vi "参数配置表.vi"() -> ()   [LabVIEW 2016, in "数据传输系统.lvlib"]
uses:
  <vilib>/Utility/miscctls.llb/LVPointTypeDef.ctl
  <vilib>/ptbypt/NI_PtbyPt.lvlib
panel:
  in  "协议标准":T1(ring)
  in  "加密传输":bool
  in  "数据库类型":enum16{"Access", "SQLite"}(ring)
  in  "应用环境":T2
  in  "屏蔽维护数据":bool
  in  "数据发送延时时间/s":i32
  in  "判断数据反馈":enum16{"非严格判断", "严格判断", "不判断"}(ring)
  in  "仪器参数发送":bool
  in  "地表水/污染源":bool
  in  "间隔时间/分钟":i32
  in  "数据发送通道":enum16{"TCP", "VISA"}(ring)
  in  "数据发送协议":enum16{"2005-212协议", "2017-212协议"}(ring)=enum."2017-212协议"
  in  "数据触发上传方式":enum16{"出数即刻发送", "间隔时间发送", "整点发送"}(ring)
  in  "数据组合发送":bool
  in  "日志、参数发送":bool
  in  "2011发送":bool
  in  "返回":bool
  out "配置表格":string[][](table)
  in  "参数数值":T3={"CODMn"=TRUE, "CODCr"=TRUE, "DO"=TRUE, "铜"=TRUE, "PH"=TRUE, "氨氮"=TRUE, "比电导率"=TRUE, "水温"=TRUE, "COD"=TRUE, "浊度"=TRUE, "总氮"=TRUE, "总磷"=TRUE, "叶绿素a"=TRUE, "藻密度"=TRUE, "水位"=TRUE, "流速"=TRUE, "瞬时流量"=TRUE, "累积流量"=TRUE, "亚硝氮"=TRUE, "硫化物"=TRUE, "ORP"=TRUE, "铅"=TRUE, "镉"=TRUE, "锌"=TRUE, "镍"=TRUE, "锰"=TRUE, "汞"=TRUE, "气温"=TRUE, "气压"=TRUE, "风速"=TRUE, "风向"=TRUE, "盐度"=TRUE, "磷酸盐"=TRUE, "硝氮"=TRUE, "氟化物"=TRUE, "挥发酚"=TRUE, "氯化物"=TRUE, "蓝绿藻"=TRUE}
  # "因子编码，单位配置，上传功能码，小时、质控数据上传触发方式"
  # "参数配置"
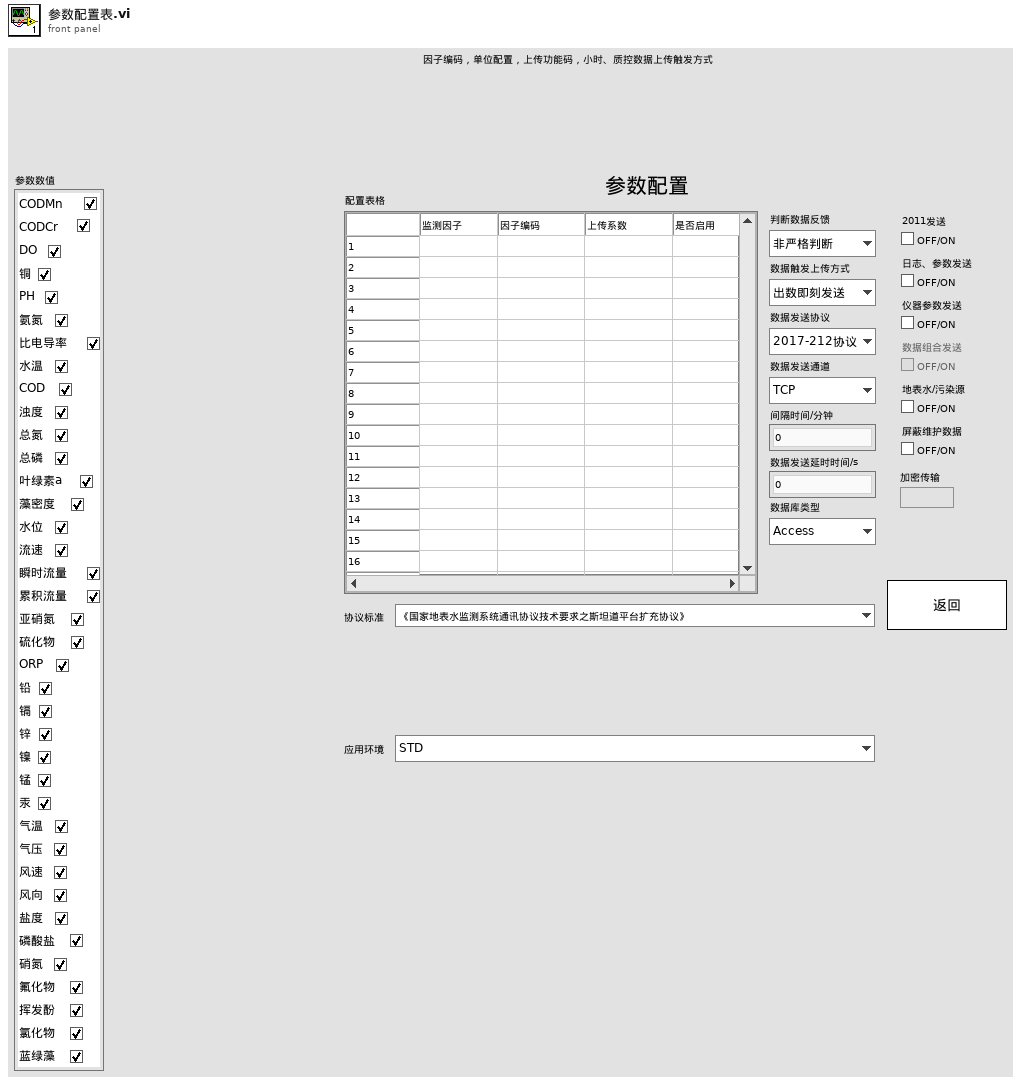
[diagram p1: front panel]
types:
  T1 = enum16{"《国家地表水监测系统通讯协议技术要求之斯坦道平台扩充协议》", "《国家地表水监测系统通讯协议技术要求》", "《国家地表水监测系统通讯协议技术要求之安徽皖仪省级平台扩充协议》"}
  T2 = typedef "数据传输系统.lvlib/应用环境.ctl" = enum16{"STD", "GB212", "婉仪平台"}
  T3 = cluster{"CODMn":bool, "CODCr":bool, "DO":bool, "铜":bool, "PH":bool, "氨氮":bool, "比电导率":bool, "水温":bool, "COD":bool, "浊度":bool, "总氮":bool, "总磷":bool, "叶绿素a":bool, "藻密度":bool, "水位":bool, "流速":bool, "瞬时流量":bool, "累积流量":bool, "亚硝氮":bool, "硫化物":bool, "ORP":bool, "铅":bool, "镉":bool, "锌":bool, "镍":bool, "锰":bool, "汞":bool, "气温":bool, "气压":bool, "风速":bool, "风向":bool, "盐度":bool, "磷酸盐":bool, "硝氮":bool, "氟化物":bool, "挥发酚":bool, "氯化物":bool, "蓝绿藻":bool}
  T4 = typedef "LVPointTypeDef.ctl" = cluster{"Horizontal":i16, "Vertical":i16}
  T5 = cluster{"[0]":string, "[1]":string, "[2]":string, "[3]":string, "[4]":string, "[5]":string, "[6]":string, "[7]":string, "[8]":string, "[9]":string, "[10]":string, "[11]":string, "[12]":string, "[13]":string, "[14]":string, "[15]":string, "[16]":string, "[17]":string, "[18]":string, "[19]":string, "[20]":string, "[21]":string, "[22]":string, "[23]":string, "[24]":string, "[25]":string, "[26]":string, "[27]":string, "[28]":string, "[29]":string, "[30]":string, "[31]":string, "[32]":string, "[33]":string, "[34]":string, "[35]":string, "[36]":string, "[37]":string}
  T6 = enum8{"Enabled", "Disabled", "Disabled and Grayed Out"}
  T7 = typedef "LVRowAndColumnTypeDef.ctl" = cluster{"Row":i32, "Column":i32}
  T8 = cluster{"[0]":string, "[1]":string, "[2]":string, "[3]":string, "[4]":string, "[5]":string, "[6]":string, "[7]":string}
  T9 = cluster{"[0]":string, "[1]":string, "[2]":string, "[3]":string, "[4]":string, "[5]":string, "[6]":string, "[7]":string, "[8]":string, "[9]":string, "[10]":string, "[11]":string, "[12]":string, "[13]":string}
  T10 = cluster{"[0]":string, "[1]":string, "[2]":string, "[3]":string, "[4]":string, "[5]":string, "[6]":string, "[7]":string, "[8]":string, "[9]":string, "[10]":string, "[11]":string, "[12]":string, "[13]":string, "[14]":string}
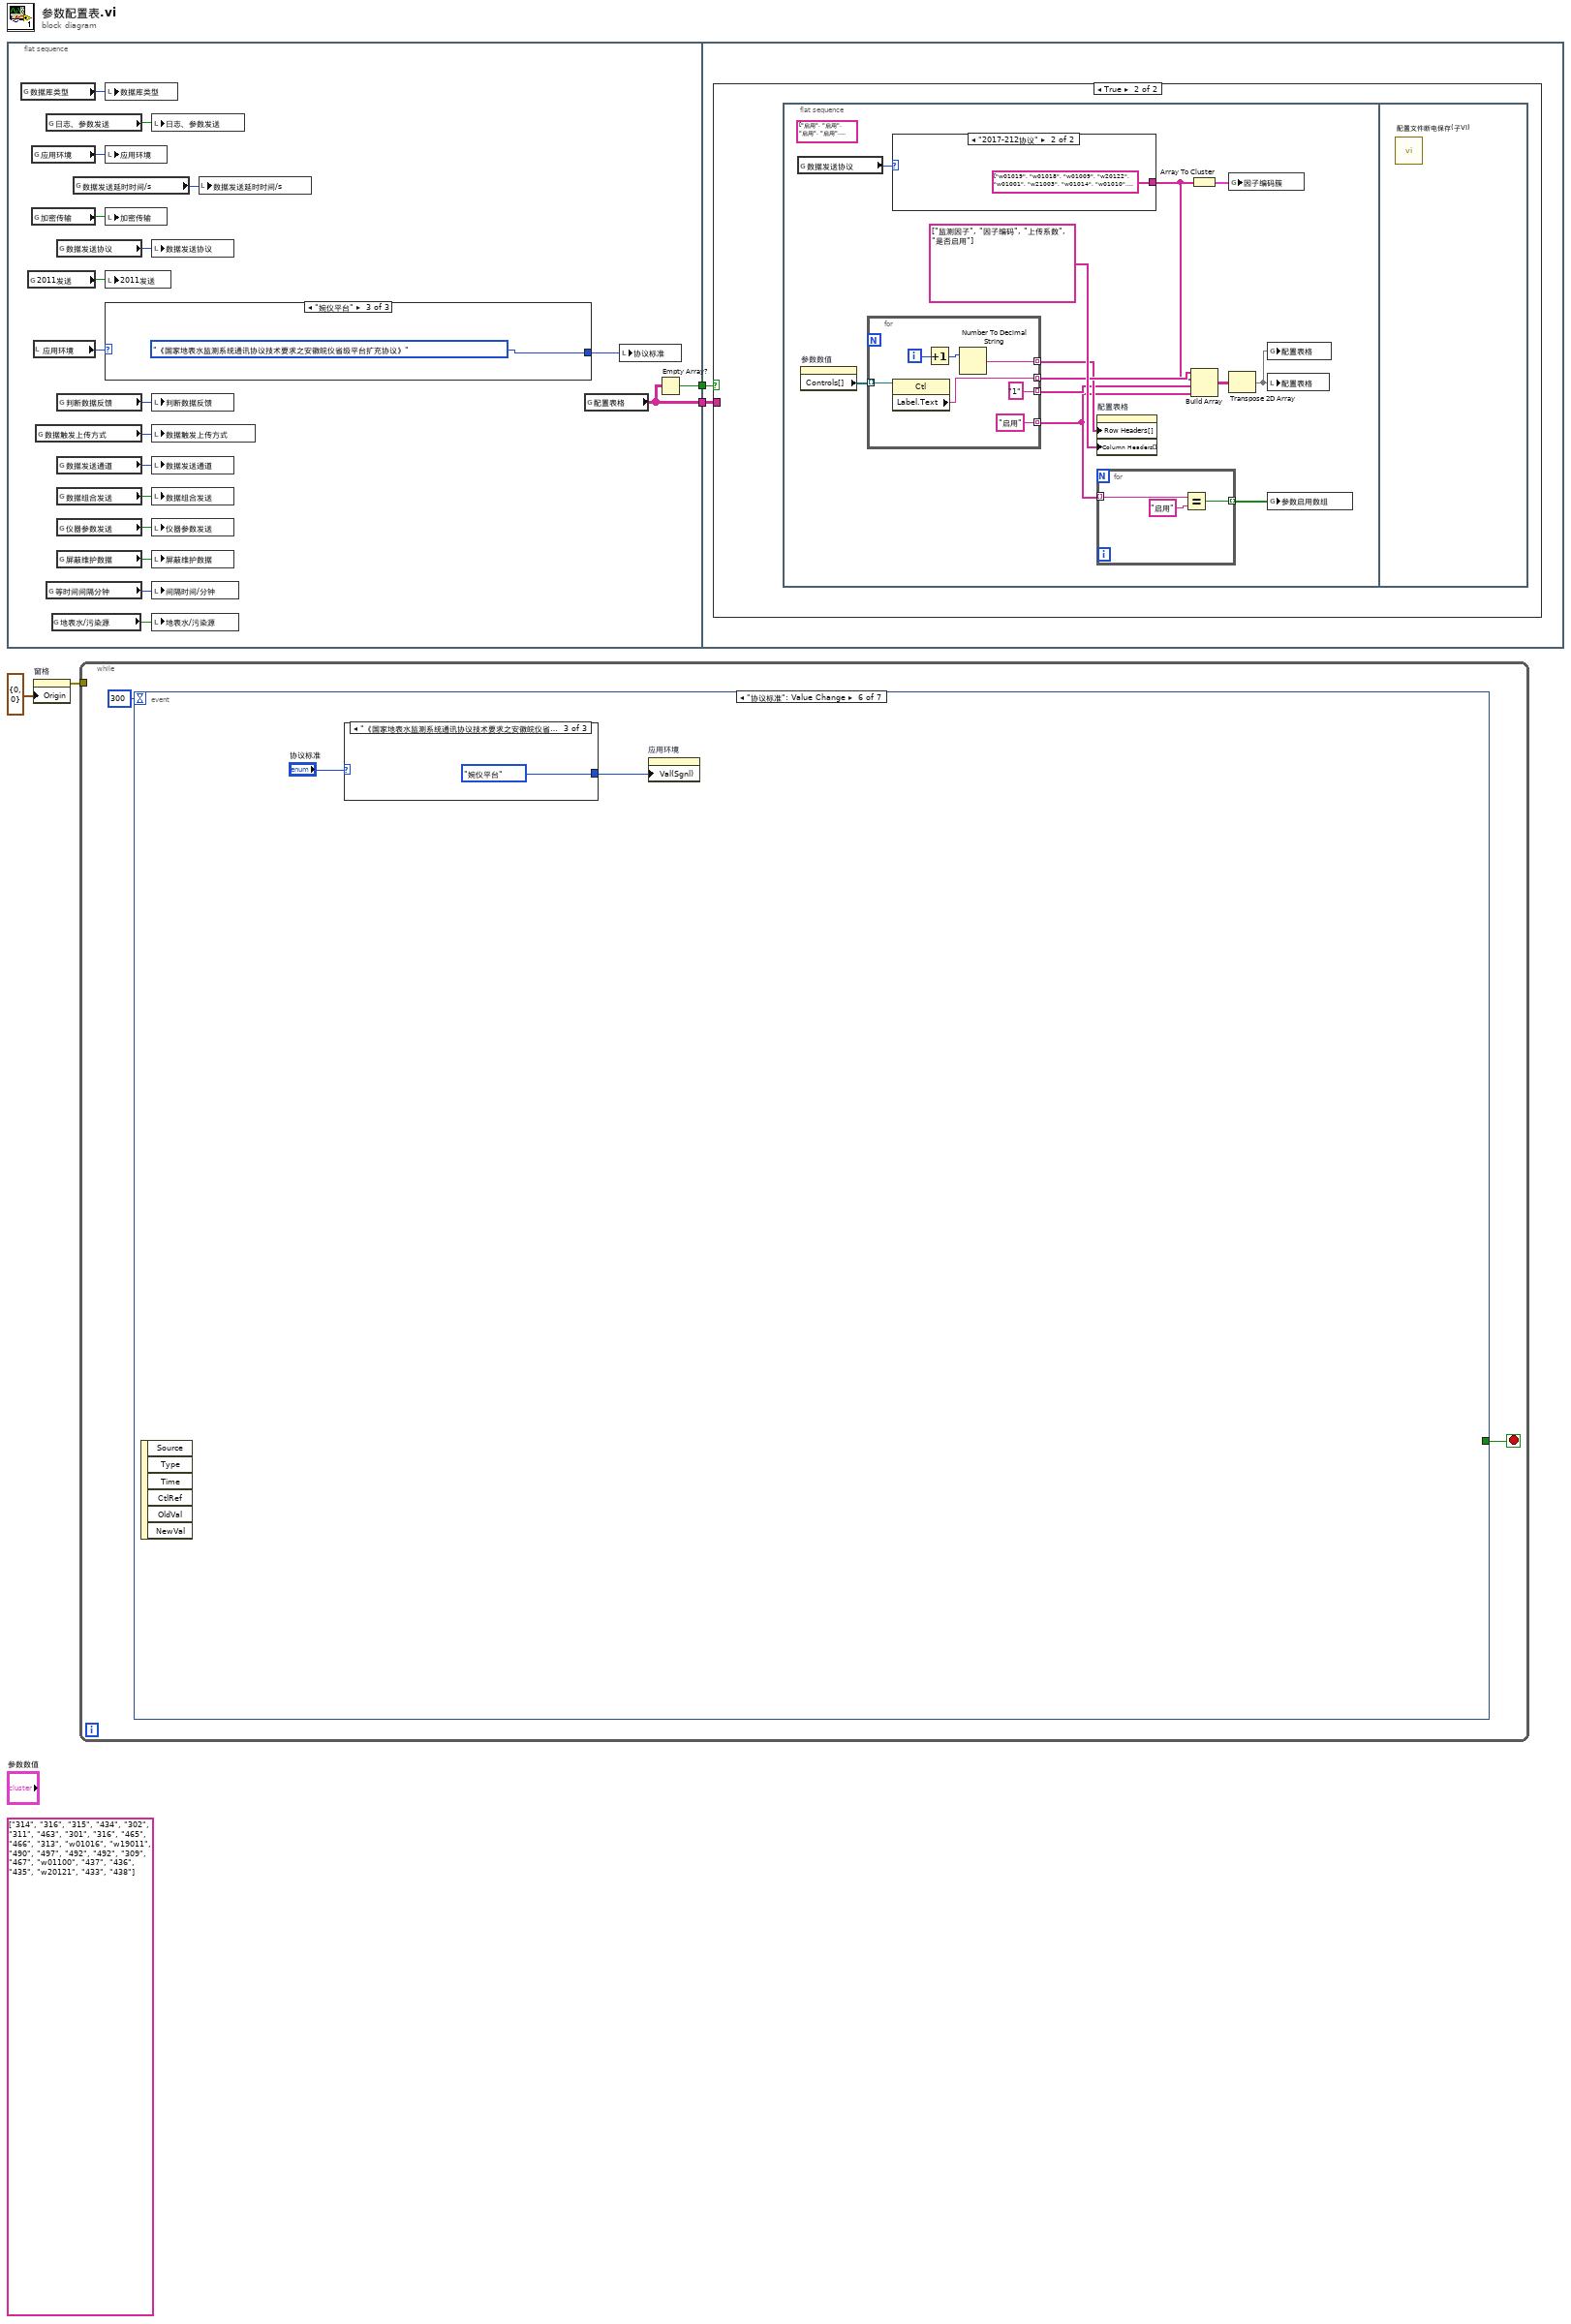
[diagram p0: block diagram]
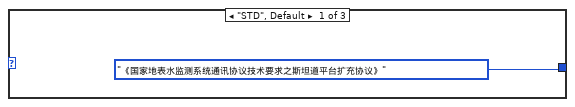
[diagram p2: hidden frame]
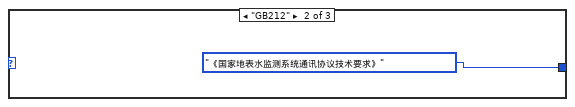
[diagram p3: hidden frame]
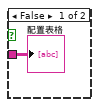
[diagram p4: hidden frame]
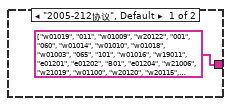
[diagram p5: hidden frame]
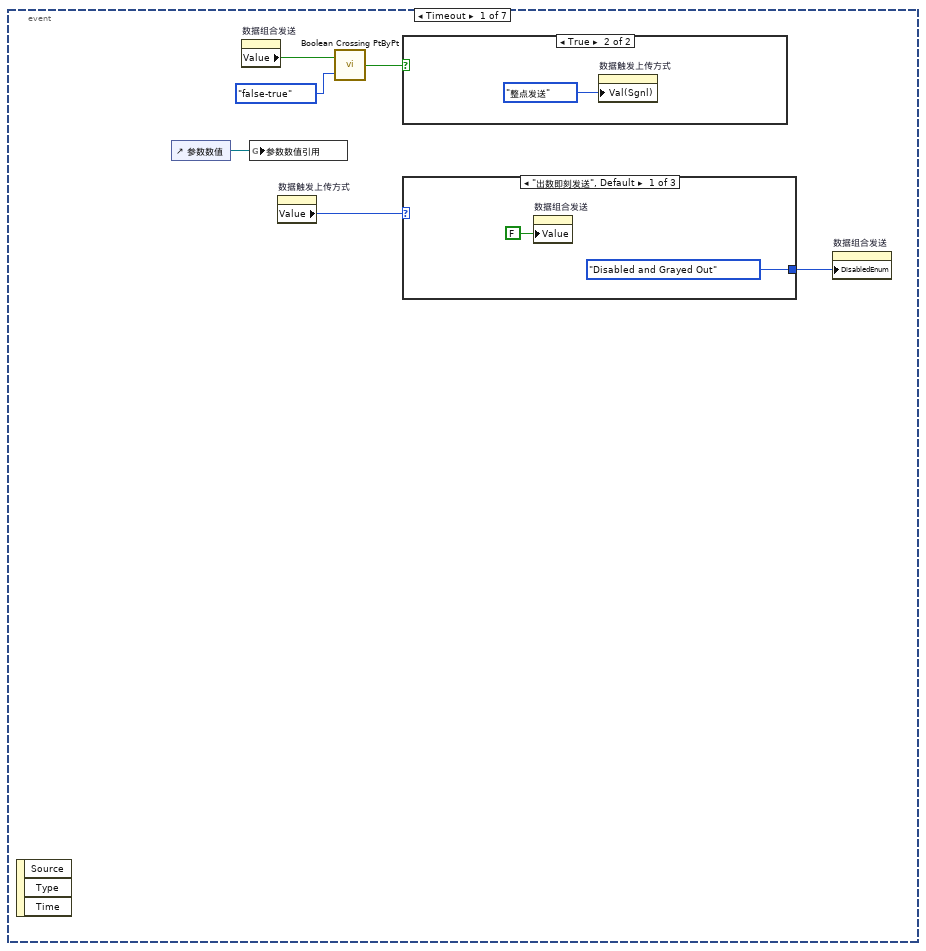
[diagram p6: hidden frame]
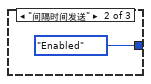
[diagram p8: hidden frame]
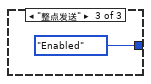
[diagram p9: hidden frame]
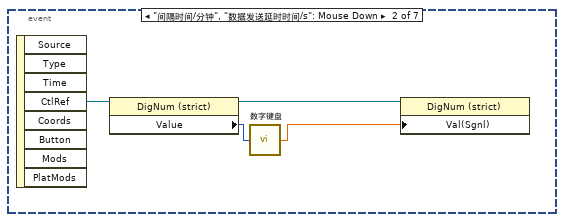
[diagram p10: hidden frame]
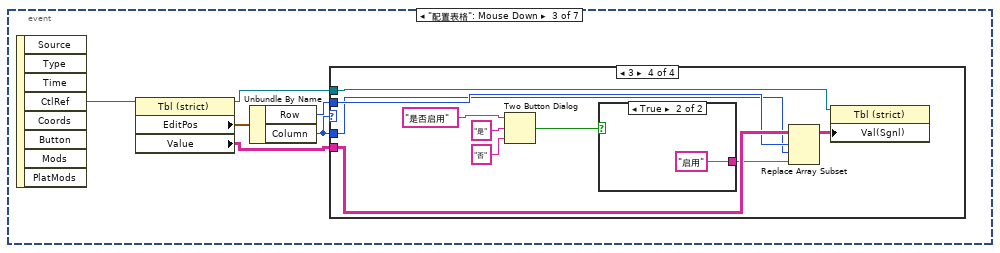
[diagram p11: hidden frame]
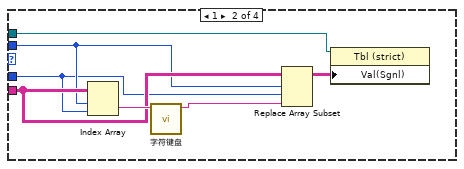
[diagram p13: hidden frame]
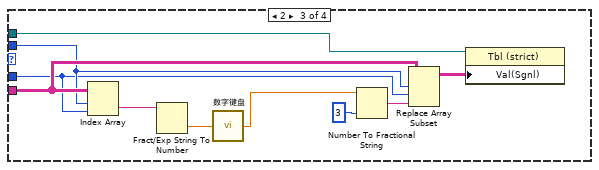
[diagram p14: hidden frame]
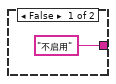
[diagram p15: hidden frame]
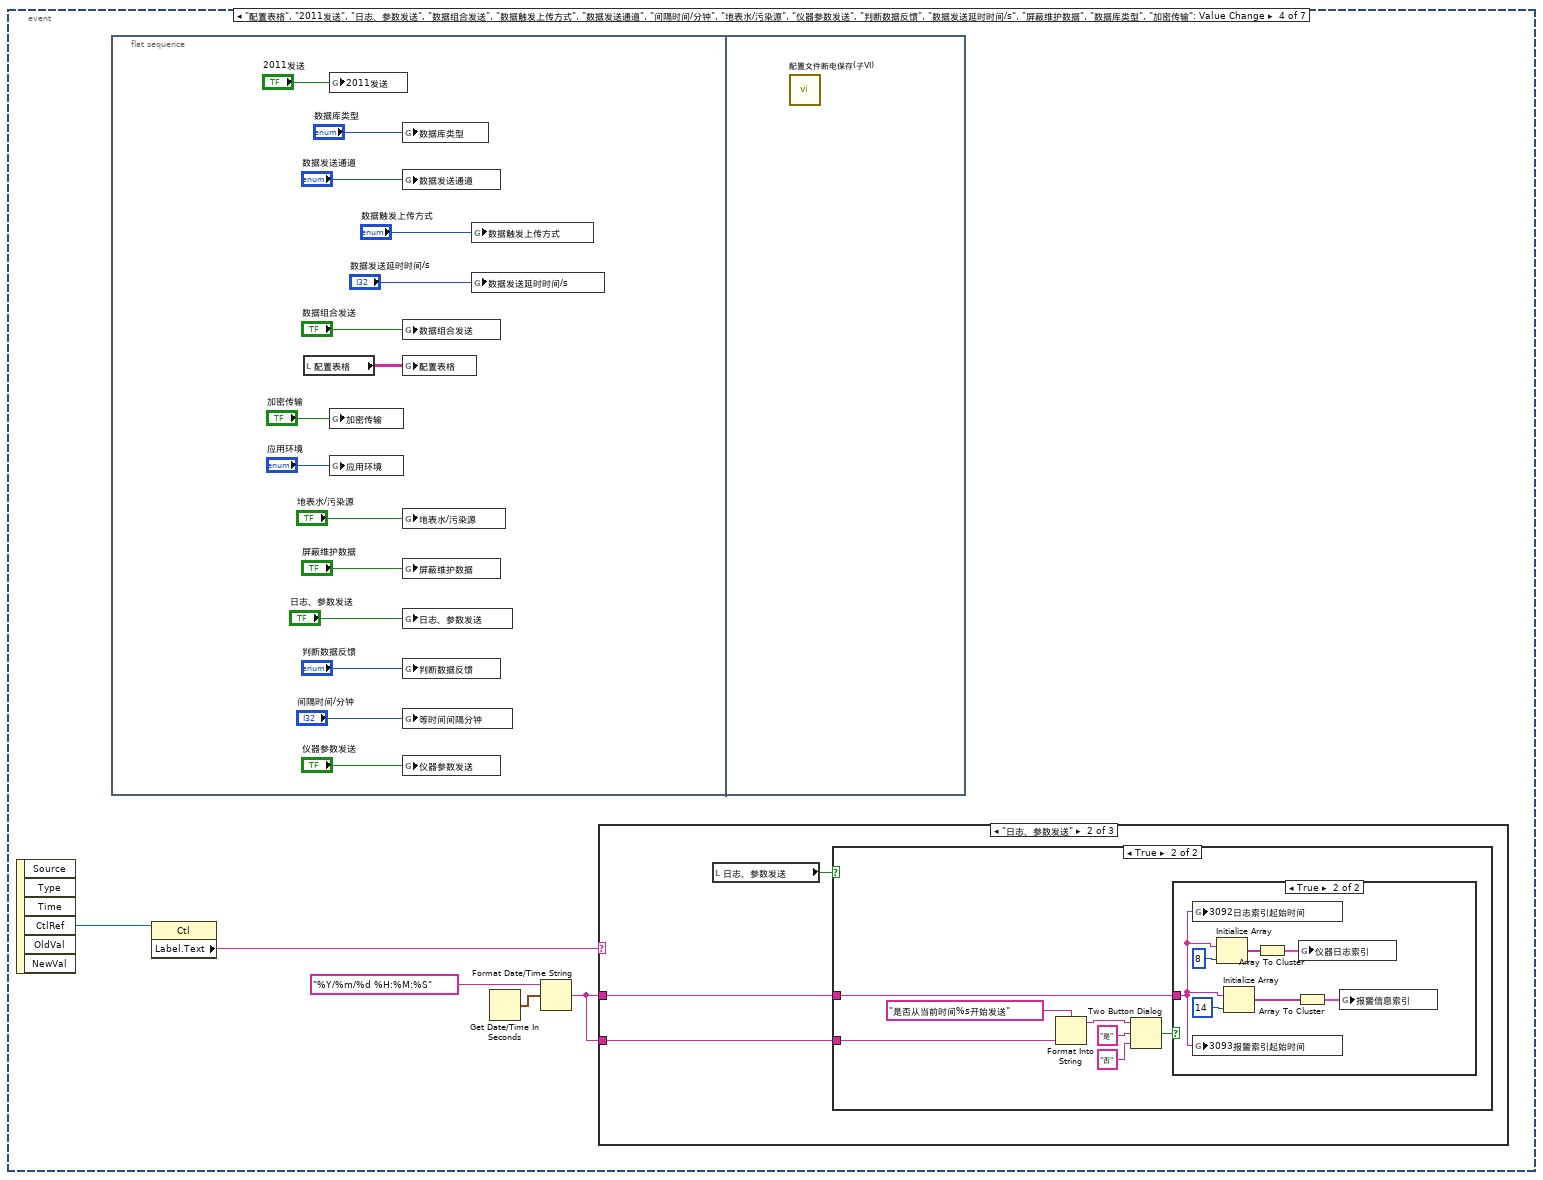
[diagram p16: hidden frame]
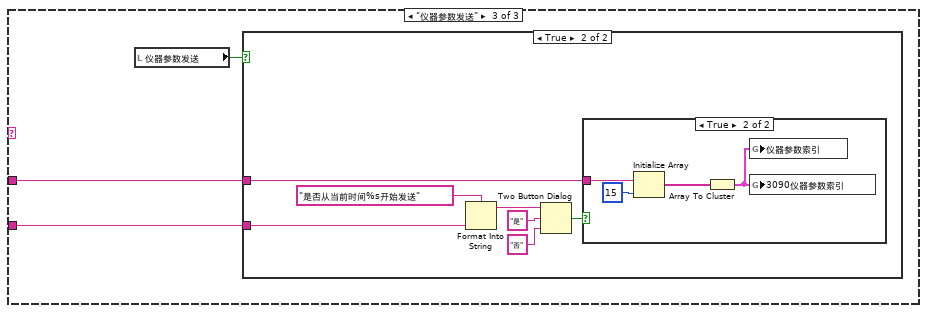
[diagram p20: hidden frame]
diagram:
  (unwired) string[] ["314", "316", "315", "434", "302", "311", "463", "301", "316", "465", "466", "313", "w01016", "w19011", "490", "497", "492", "492", "309", "467", "w01100", "437", "436", "435", "w20121", "433", "438"]
  n1 = flat-sequence {
    tunnel: [w16] -> w2
    tunnel: [w15] -> w1
    tunnel: w2 -> [w28]
    tunnel: w1 -> [w27]
    frame #0 {
      n2 = global read "断电保存全局.vi" "数据库类型"() -> (w8:enum16{"Access", "SQLite"})
      n3 = global read "断电保存全局.vi" "2011发送"() -> (w23:bool)
      n4 = global read "断电保存全局.vi" "应用环境"() -> (w9:T2)
      n5 = global read "断电保存全局.vi" "加密传输"() -> (w7:bool)
      n6 = local read "应用环境"() -> (w6:T2)
      n7 = global read "断电保存全局.vi" "数据触发上传方式"() -> (w19:enum16{"出数即刻发送", "间隔时间发送", "整点发送"})
      n8 = global read "断电保存全局.vi" "日志、参数发送"() -> (w21:bool)
      n9 = global read "断电保存全局.vi" "等时间间隔分钟"() -> (w14:i32)
      n10 = global read "断电保存全局.vi" "地表水/污染源"() -> (w13:bool)
      n11 = global read "断电保存全局.vi" "数据发送协议"() -> (w17:enum16{"2005-212协议", "2017-212协议"})
      n12 = global read "断电保存全局.vi" "判断数据反馈"() -> (w22:enum16{"非严格判断", "严格判断", "不判断"})
      n13 = global read "断电保存全局.vi" "数据发送通道"() -> (w18:enum16{"TCP", "VISA"})
      n14 = global read "断电保存全局.vi" "数据组合发送"() -> (w20:bool)
      n15 = global read "断电保存全局.vi" "仪器参数发送"() -> (w12:bool)
      n16 = global read "断电保存全局.vi" "屏蔽维护数据"() -> (w10:bool)
      n17 = global read "断电保存全局.vi" "数据发送延时时间/s"() -> (w11:i32)
      n18 = local write "数据库类型"(w8) -> ()
      n19 = local write "应用环境"(w9) -> ()
      n20 = local write "加密传输"(w7) -> ()
      n21 = local write "2011发送"(w23) -> ()
      n22 = case shown="\"婉仪平台\"" w6 {
        tunnel: [T1."《国家地表水监测系统通讯协议技术要求之斯坦道平台扩充协议》" ("协议标准") T1."《国家地表水监测系统通讯协议技术要求》" ("协议标准") T1."《国家地表水监测系统通讯协议技术要求之安徽皖仪省级平台扩充协议》" ("协议标准")] -> w5
        frame "STD", Default {
        }
        frame "GB212" {
        }
        frame "婉仪平台" {
        }
      }
      n23 = local write "日志、参数发送"(w21) -> ()
      n24 = local write "数据发送协议"(w17) -> ()
      n25 = local write "判断数据反馈"(w22) -> ()
      n26 = local write "数据触发上传方式"(w19) -> ()
      n27 = local write "数据发送通道"(w18) -> ()
      n28 = local write "数据组合发送"(w20) -> ()
      n29 = local write "仪器参数发送"(w12) -> ()
      n30 = local write "屏蔽维护数据"(w10) -> ()
      n31 = local write "间隔时间/分钟"(w14) -> ()
      n32 = local write "地表水/污染源"(w13) -> ()
      n33 = local write "数据发送延时时间/s"(w11) -> ()
      n34 = global read "断电保存全局.vi" "配置表格"() -> (w15:string[][])
      n35 = local write "协议标准"(w5) -> ()
      n36 = Empty Array?(array=w15) -> (empty?=w16:bool)
    }
    frame #1 {
      n37 = case shown="True" w28 {
        tunnel: w27 -> [w29 _]
        frame False {
          "配置表格" <- w29
        }
        frame True {
          n38 = flat-sequence {
            frame #0 {
              (unwired) string[] ["启用", "启用", "启用", "启用", "启用", "启用", "启用", "启用", "启用", "启用", "启用", "启用", "启用", "启用", "启用", "启用", "启用", "启用", "启用", "启用", "启用", "启用", "启用", "启用", "启用", "启用", "启用"]
              n39 = global read "断电保存全局.vi" "数据发送协议"() -> (w31:enum16{"2005-212协议", "2017-212协议"})
              n40 = property on="参数数值" class="Clust (strict)"() -> ("Controls[]"=w37:refnum<vi>[])  [unwired: 2 in, 2 out]
              n41 = for {
                tunnel: w37 -> [w53] mode=indexing
                tunnel: [w52] -> w39 mode=indexing
                tunnel: [w50] -> w38 mode=indexing
                tunnel: ["1"] -> w34 mode=indexing
                tunnel: ["启用"] -> w32 mode=indexing
                i -> [w51]
                n42 = property class="Ctl"(reference=w53) -> ("Label.Text"=w52:string)  [unwired: 1 in, 2 out]
                n43 = Increment(x=w51) -> (x+1=w49:i32)
                n44 = Number To Decimal String(number=w49) -> (decimal integer string=w50:string)  [unwired: 1 in]
              }
              n45 = case shown="\"2017-212协议\"" w31 {
                tunnel: [string[] ["w01019", "011", "w01009", "w20122", "001", "060", "w01014", "w01010", "w01018", "w01003", "065", "101", "w01016", "w19011", "e01201", "e01202", "B01", "e01204", "w21006", "w21019", "w01100", "w20120", "w20115", "w20123", "w20121", "w20124", "w20111", "a01001", "a01006", "a01007", "a01008", "w01002", "w21015", "w21007", "w21017", "w23002", "w21002", "w01022"] string[] ["w01019", "w01018", "w01009", "w20122", "w01001", "w21003", "w01014", "w01010", "w01018", "w01003", "w21001", "w21011", "w01016", "w19011", "e01201", "e01202", "e01203", "e01204", "w21006", "w21019", "w01100", "w20120", "w20115", "w20123", "w20121", "w20124", "w20111", "a01001", "a01006", "a01007", "a01008", "w01002", "w21015", "w21007", "w21017", "w23002", "w21002", "w01022"]] -> w30
                frame "2005-212协议", Default {
                }
                frame "2017-212协议" {
                }
              }
              n46 = property on="配置表格" class="Tbl (strict)"("Row Headers[]"=w38, "Column Headers[]"=string[] ["监测因子", "因子编码", "上传系数", "是否启用"]) -> ()  [unwired: 2 in, 2 out]
              n47 = for {
                tunnel: w32 -> [w46] mode=indexing
                tunnel: [w44] -> w33 mode=indexing
                n48 = Equal?(x=w46, y="启用") -> (x = y?=w44:bool)
              }
              n49 = Array To Cluster(array=w30) -> (cluster=w35:T5)
              n50 = Build Array(w39, w30, w34, w32) -> (w41:string[][])
              n51 = global write "断电保存全局.vi" "因子编码簇"(w35) -> ()
              n52 = Transpose 2D Array(2D array=w41) -> (transposed array=w36:string[][])
              n53 = global write "断电保存全局.vi" "配置表格"(w36) -> ()
              n54 = local write "配置表格"(w36) -> ()
              n55 = global write "断电保存全局.vi" "参数启用数组"(w33) -> ()
            }
            frame #1 {
              n56 = call "配置文件断电保存(子VI).vi"() -> ()  [unwired: 12 in]
            }
          }
        }
      }
    }
  }
  n57 = property on="窗格" class="Pane"("Origin"=T4 {"Horizontal"=0, "Vertical"=0} ("原点")) -> (error out=w4:errorcluster)  [unwired: 2 in, 1 out]
  n58 = while {
    tunnel: w4 -> [_]
    stop <- w54 stop-if-true
    n59 = event shown="[5] \"协议标准\": Value Change" {
      selector: _ -> [_ _ _ _ _ _ _]
      dyn-events: _ -> [_ _ _ _ _ _ _]
      timeout: 300 -> [_ _ _ _ _ _ _]
      tunnel: [_ _ _ _ _ _ TRUE] -> w54
      event Timeout {
        n60 = event-data() -> ()  [unwired: 1 in, 3 out]
        n61 = control-ref of="参数数值"() -> (w56:refnum<vi>)
        n62 = property on="数据组合发送" class="Bool (strict)"() -> ("Value"=w59:bool)  [unwired: 2 in, 2 out]
        n63 = global write "断电保存全局.vi" "参数数值引用"(w56) -> ()
        n64 = property on="数据触发上传方式" class="Enum (strict)"() -> ("Value"=w61:enum16{"出数即刻发送", "间隔时间发送", "整点发送"})  [unwired: 2 in, 2 out]
        n65 = call <vilib>:"Boolean Crossing PtByPt.vi"("direction"=enum16{"either", "false-true", "true-false"}."false-true", "input"=w59) -> ("crossing"=w57:bool)  [unwired: 1 in]
        n66 = case shown="True" w57 {
          frame False {
          }
          frame True {
            n67 = property on="数据触发上传方式" class="Enum (strict)"("Val(Sgnl)"=enum16{"出数即刻发送", "间隔时间发送", "整点发送"}."整点发送" ("值(信号)")) -> ()  [unwired: 2 in, 2 out]
          }
        }
        n68 = case shown="\"出数即刻发送\", Default" w61 {
          tunnel: [T6."Disabled and Grayed Out" ("禁用") T6."Enabled" ("禁用") T6."Enabled" ("禁用")] -> w60
          frame "出数即刻发送", Default {
            n69 = property on="数据组合发送" class="Bool (strict)"("Value"=FALSE ("值(信号)")) -> ()  [unwired: 2 in, 2 out]
          }
          frame "间隔时间发送" {
          }
          frame "整点发送" {
          }
        }
        n70 = property on="数据组合发送" class="Bool (strict)"("DisabledEnum"=w60) -> ()  [unwired: 2 in, 2 out]
      }
      event "间隔时间/分钟", "数据发送延时时间/s": Mouse Down {
        n71 = event-data() -> ("CtlRef"=w70:refnum<vi>)  [unwired: 1 in, 7 out]
        n72 = property class="DigNum (strict)"(reference=w70) -> (reference out=w68:refnum<vi>, "Value"=w69:i32)  [unwired: 1 in, 1 out]
        n73 = call "数字键盘.vi"("OldNumber"=w69) -> ("NewNumber"=w67:sgl)
        n74 = property class="DigNum (strict)"(reference=w68, "Val(Sgnl)"=w67) -> ()  [unwired: 1 in, 2 out]
      }
      event "配置表格": Mouse Down {
        n75 = event-data() -> ("CtlRef"=w76:refnum<vi>)  [unwired: 1 in, 7 out]
        n76 = property class="Tbl (strict)"(reference=w76) -> (reference out=w72:refnum<vi>, "EditPos"=w75:T7, "Value"=w74:string[][])  [unwired: 1 in, 1 out]
        n77 = Unbundle By Name(w75) -> ("Row"=w73:i32, "Column"=w71:i32)
        n78 = case shown="3" w71 {
          tunnel: w74 -> [_ w82 w93 w97]
          tunnel: w73 -> [_ w81 w92 w96]
          tunnel: w71 -> [_ w80 w91 w95]
          tunnel: w72 -> [_ w78 w90 w98]
          frame 0, Default {
          }
          frame 1 {
            n79 = Index Array(array=w82, index (row)=w81, index (col)=w80) -> (element=w83:string)
            n80 = call "字符键盘.vi"("原值"=w83) -> ("x+y"=w79:string)  [unwired: 10 in]
            n81 = Replace Array Subset(array=w82, new element=w79, index (row)=w81, index (col)=w80) -> (w77:string[][])
            n82 = property class="Tbl (strict)"(reference=w78, "Val(Sgnl)"=w77) -> ()  [unwired: 1 in, 2 out]
          }
          frame 2 {
            n83 = Index Array(array=w93, index (row)=w92, index (col)=w91) -> (element=w88:string)
            n84 = Fract/Exp String To Number(string=w88) -> (number=w87:dbl)  [unwired: 3 in, 1 out]
            n85 = call "数字键盘.vi"("OldNumber"=w87) -> ("NewNumber"=w86:sgl)
            n86 = Number To Fractional String(number=w86, precision (6)=i16 3 ("精度(6)")) -> (F-format string=w85:string)  [unwired: 2 in]
            n87 = Replace Array Subset(array=w93, new element=w85, index (row)=w92, index (col)=w91) -> (w89:string[][])
            n88 = property class="Tbl (strict)"(reference=w90, "Val(Sgnl)"=w89) -> ()  [unwired: 1 in, 2 out]
          }
          frame 3 {
            n89 = Two Button Dialog(message="是否启用" ("消息"), 1:"否" ("F按钮名称（“取消”）"), 2:"是" ("T按钮名称（“确定”）")) -> (T button?=w100:bool)
            n90 = case shown="True" w100 {
              tunnel: ["不启用" "启用"] -> w94
              frame False {
              }
              frame True {
              }
            }
            n91 = Replace Array Subset(array=w97, new element=w94, index (row)=w96, index (col)=w95) -> (w99:string[][])
            n92 = property class="Tbl (strict)"(reference=w98, "Val(Sgnl)"=w99) -> ()  [unwired: 1 in, 2 out]
          }
        }
      }
      event "配置表格", "2011发送", "日志、参数发送", "数据组合发送", "数据触发上传方式", "数据发送通道", "间隔时间/分钟", "地表水/污染源", "仪器参数发送", "判断数据反馈", "数据发送延时时间/s", "屏蔽维护数据", "数据库类型", "加密传输": Value Change {
        n93 = event-data() -> ("CtlRef"=w110:refnum<vi>)  [unwired: 1 in, 5 out]
        n94 = flat-sequence {
          frame #0 {
            n95 = local read "配置表格"() -> (w156:string[][])
            n96 = global write "断电保存全局.vi" "2011发送"("2011发送") -> ()
            n97 = global write "断电保存全局.vi" "加密传输"("加密传输") -> ()
            n98 = global write "断电保存全局.vi" "应用环境"("应用环境") -> ()
            n99 = global write "断电保存全局.vi" "数据库类型"("数据库类型") -> ()
            n100 = global write "断电保存全局.vi" "数据发送通道"("数据发送通道") -> ()
            n101 = global write "断电保存全局.vi" "数据组合发送"("数据组合发送") -> ()
            n102 = global write "断电保存全局.vi" "配置表格"(w156) -> ()
            n103 = global write "断电保存全局.vi" "地表水/污染源"("地表水/污染源") -> ()
            n104 = global write "断电保存全局.vi" "屏蔽维护数据"("屏蔽维护数据") -> ()
            n105 = global write "断电保存全局.vi" "日志、参数发送"("日志、参数发送") -> ()
            n106 = global write "断电保存全局.vi" "判断数据反馈"("判断数据反馈") -> ()
            n107 = global write "断电保存全局.vi" "等时间间隔分钟"("间隔时间/分钟") -> ()
            n108 = global write "断电保存全局.vi" "仪器参数发送"("仪器参数发送") -> ()
            n109 = global write "断电保存全局.vi" "数据触发上传方式"("数据触发上传方式") -> ()
            n110 = global write "断电保存全局.vi" "数据发送延时时间/s"("数据发送延时时间/s") -> ()
          }
          frame #1 {
            n111 = call "配置文件断电保存(子VI).vi"() -> ()  [unwired: 12 in]
          }
        }
        n112 = property class="Ctl"(reference=w110) -> ("Label.Text"=w109:string)  [unwired: 1 in, 2 out]
        n113 = Get Date/Time In Seconds() -> (seconds since 1Jan1904=w108:timestamp)
        n114 = Format Date/Time String(time format string (%c)="%Y/%m/%d %H:%M:%S" ("时间格式字符串(%c)"), seconds (now)=w108) -> (date/time string=w106:string)  [unwired: 1 in]
        n115 = case shown="\"日志、参数发送\"" w109 {
          tunnel: w106 -> [_ w112 w129]
          tunnel: w106 -> [_ w111 w128]
          frame "假", Default {
          }
          frame "日志、参数发送" {
            n116 = local read "日志、参数发送"() -> (w113:bool)
            n117 = case shown="True" w113 {
              tunnel: w112 -> [_ w117]
              tunnel: w111 -> [_ w115]
              frame False {
              }
              frame True {
                n118 = Format Into String(format string="是否从当前时间%s开始发送" ("消息"), w115) -> (resulting string=w114:string)  [unwired: 2 in, 1 out]
                n119 = Two Button Dialog(message=w114, 1:"否" ("F按钮名称（“取消”）"), 2:"是" ("T按钮名称（“确定”）")) -> (T button?=w118:bool)
                n120 = case shown="True" w118 {
                  tunnel: w117 -> [_ w121]
                  frame False {
                  }
                  frame True {
                    n121 = global write "全局 时间2.vi" "3092日志索引起始时间"(w121) -> ()
                    n122 = global write "全局 时间2.vi" "3093报警索引起始时间"(w121) -> ()
                    n123 = Initialize Array(w121, 8 ("维数大小")) -> (w122:string[])
                    n124 = Initialize Array(w121, 14 ("维数大小")) -> (w125:string[])
                    n125 = Array To Cluster(array=w122) -> (cluster=w123:T8)
                    n126 = Array To Cluster(array=w125) -> (cluster=w124:T9)
                    n127 = global write "全局 时间2.vi" "仪器日志索引"(w123) -> ()
                    n128 = global write "全局 时间2.vi" "报警信息索引"(w124) -> ()
                  }
                }
              }
            }
          }
          frame "仪器参数发送" {
            n129 = local read "仪器参数发送"() -> (w130:bool)
            n130 = case shown="True" w130 {
              tunnel: w129 -> [_ w134]
              tunnel: w128 -> [_ w132]
              frame False {
              }
              frame True {
                n131 = Format Into String(format string="是否从当前时间%s开始发送" ("消息"), w132) -> (resulting string=w131:string)  [unwired: 2 in, 1 out]
                n132 = Two Button Dialog(message=w131, 1:"否" ("F按钮名称（“取消”）"), 2:"是" ("T按钮名称（“确定”）")) -> (T button?=w135:bool)
                n133 = case shown="True" w135 {
                  tunnel: w134 -> [_ w139]
                  frame False {
                  }
                  frame True {
                    n134 = Initialize Array(w139, 15 ("维数大小")) -> (w141:string[])
                    n135 = Array To Cluster(array=w141) -> (cluster=w138:T10)
                    n136 = global write "全局 时间2.vi" "仪器参数索引"(w138) -> ()
                    n137 = global write "全局 时间2.vi" "3090仪器参数索引"(w138) -> ()
                  }
                }
              }
            }
          }
        }
      }
      event "数据发送协议": Value Change {
        n138 = event-data() -> ()  [unwired: 1 in, 6 out]
        n139 = flat-sequence {
          frame #0 {
            n140 = global write "断电保存全局.vi" "数据发送协议"("数据发送协议") -> ()
            n141 = case shown="\"2017-212协议\"" "数据发送协议" {
              tunnel: [string[] ["w01019", "011", "w01009", "w20122", "001", "060", "w01014", "w01010", "w01018", "w01003", "065", "101", "w01016", "w19011", "e01201", "e01202", "B01", "e01204", "w21006", "w21019", "w01100", "w20120", "w20115", "w20123", "w20121", "w20124", "w20111", "a01001", "a01006", "a01007", "a01008", "w01002", "w21015", "w21007", "w21017", "w23002", "w21002", "w01022"] string[] ["w01019", "w01018", "w01009", "w20122", "w01001", "w21003", "w01014", "w01010", "w01018", "w01003", "w21001", "w21011", "w01016", "w19011", "e01201", "e01202", "e01203", "e01204", "w21006", "w21019", "w01100", "w20120", "w20115", "w20123", "w20121", "w20124", "w20111", "a01001", "a01006", "a01007", "a01008", "w01002", "w21015", "w21007", "w21017", "w23002", "w21002", "w01022"]] -> w157
              frame "2005-212协议", Default {
              }
              frame "2017-212协议" {
              }
            }
            n142 = local read "配置表格"() -> (w161:string[][])
            n143 = Replace Array Subset(array=w161, new element=w157, index (col)=1 ("禁用的索引 (列)")) -> (w159:string[][])  [unwired: 1 in]
            n144 = property on="配置表格" class="Tbl (strict)"("Val(Sgnl)"=w159) -> ()  [unwired: 2 in, 2 out]
            n145 = global write "断电保存全局.vi" "配置表格"(w159) -> ()
          }
          frame #1 {
            n146 = call "配置文件断电保存(子VI).vi"() -> ()  [unwired: 12 in]
          }
        }
      }
      event "协议标准": Value Change {
        n147 = event-data() -> ()  [unwired: 1 in, 6 out]
        n148 = case shown="\"《国家地表水监测系统通讯协议技术要求之安徽皖仪省级平台扩充协议》\"" "协议标准" {
          tunnel: [应用环境."STD" ("值(信号)") 应用环境."GB212" ("值(信号)") 应用环境."婉仪平台" ("值(信号)")] -> w164
          frame "《国家地表水监测系统通讯协议技术要求之斯坦道平台扩充协议》", Default {
          }
          frame "《国家地表水监测系统通讯协议技术要求》" {
          }
          frame "《国家地表水监测系统通讯协议技术要求之安徽皖仪省级平台扩充协议》" {
          }
        }
        n149 = property on="应用环境" class="Enum (strict)"("Val(Sgnl)"=w164) -> ()  [unwired: 2 in, 2 out]
      }
      event "返回": Value Change; Panel Close {
        n150 = event-data() -> ()  [unwired: 1 in, 3 out]
      }
    }
  }
